vi "ReturnNameNadChildren.vi"(8 "error in (no error)":errorcluster, 11 "Interface in":refnum<class "Interface.lvclass">) -> (0 "error out":errorcluster, 1 "Children":refnum<class "Class.lvclass">[](array[class]), 2 "Name":string, 3 "Interface out":refnum<class "Interface.lvclass">)   [LabVIEW 2020, in "Mermaid.lvlib" / "Interface.lvclass"]
uses:
  Interface.lvclass
  _Class/Class.lvclass
  Interface.lvclass/Interface.ctl
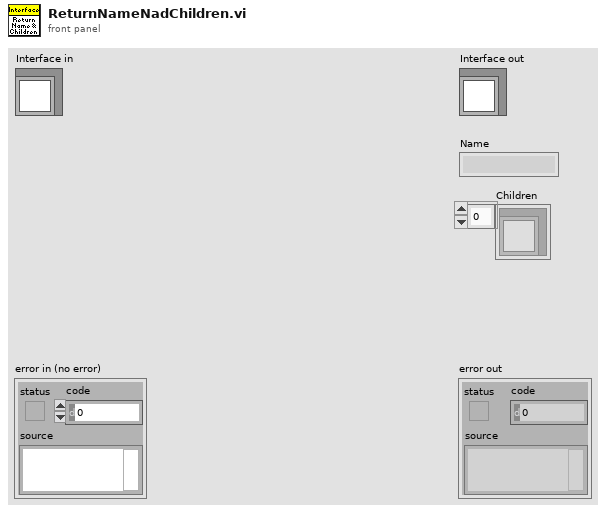
[diagram p1: front panel]
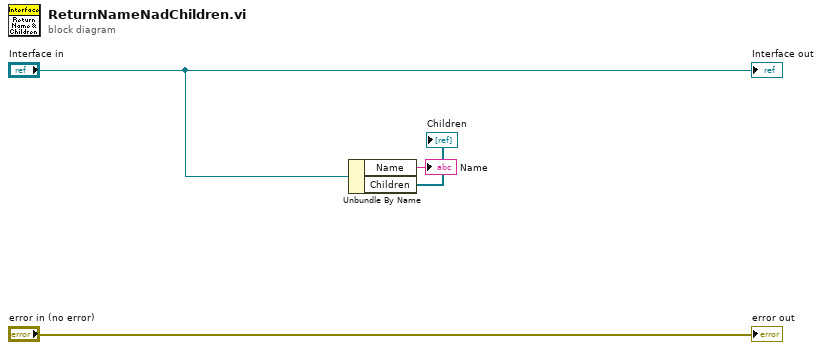
[diagram p0: block diagram]
diagram:
  n1 = Unbundle By Name("Interface in") -> ("Name"=→"Name":string, "Children"=→"Children":refnum<class "Class.lvclass">[])
  "error out" <- "error in (no error)"
  "Interface out" <- "Interface in"
